vi "BuildTestFromProjectItem_EmptyLibrary_BuildsEmptyTestSuite.vi"() -> ()   [LabVIEW 2017, in "LVUnitTestBuilderTest.lvlib"]
uses:
  LVUnitTestBuilderTest.lvlib
  LVUnitTestBuilder/LVUnitTestBuilder.lvclass
  TestSuite/TestSuite.lvclass
  a12a2084-e44a-4edc-a973-f21fdd0e5ac6.vi
panel:
  out "error out":errorcluster
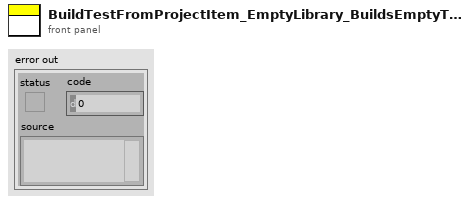
[diagram p1: front panel]
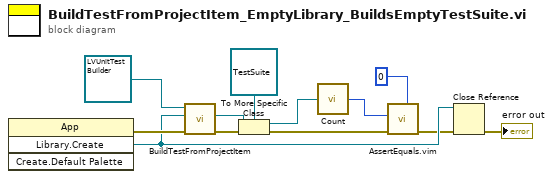
[diagram p0: block diagram]
diagram:
  n1 = invoke class="App" method="Library.Create"() -> (error out=w11:errorcluster, "Create Library"=w6:refnum<vi>)  [unwired: 4 in, 2 out]
  n2 = call-dynamic "BuildTestFromProjectItem.vi"("error in (no error)"=w11, "ProjectItem Refnum"=w6, "LVUnitTestBuilder in"=refnum<class "LVUnitTestBuilder.lvclass"> refnum ("LVUnitTestBuilder")) -> ("error out"=w5:errorcluster, "Test"=w10:refnum<class "Test.lvclass">)  [unwired: 6 in, 1 out]
  n3 = To More Specific Class(target class=refnum<class "TestSuite.lvclass"> refnum ("TestSuite.lvclass"), reference=w10, error in=w5) -> (specific class reference=w8:refnum<class "TestSuite.lvclass">, error out=w4:errorcluster)
  n4 = call "Count.vi"("TestSuite In"=w8) -> ("Count"=w2:i32)
  n5 = call "AssertEquals.vim"("Expected"=0 ("Count"), "error in (no error)"=w4, "Actual"=w2) -> ("error out"=w3:errorcluster)  [unwired: 8 in]
  n6 = Close Reference(reference=w6, error in (no error)=w3) -> (error out=→"error out":errorcluster)
